vi "Load Hardware.vi"(8 "error in (no error)":errorcluster, 10 "Program only changes":bool=TRUE, 11 "Agilent ESG in":refnum<class "Agilent ESG.lvclass">) -> (0 "error out":errorcluster, 3 "Agilent ESG out":refnum<class "Agilent ESG.lvclass">)   [LabVIEW 2013, in "Agilent ESG.lvclass"]
uses:
  Agilent ESG.lvclass
  Agilent ESG.lvclass/Agilent ESG.ctl
panel:
  out "Hardware Image.Freq. [MHz]":dbl[](array[numeric])
  out "Last HWI Array":T1(array[cluster])
  out "Names encountered":string[](array[string])
  # "encapsulate HWI in cluser so each \"last encountered\"\ncan be a different length."
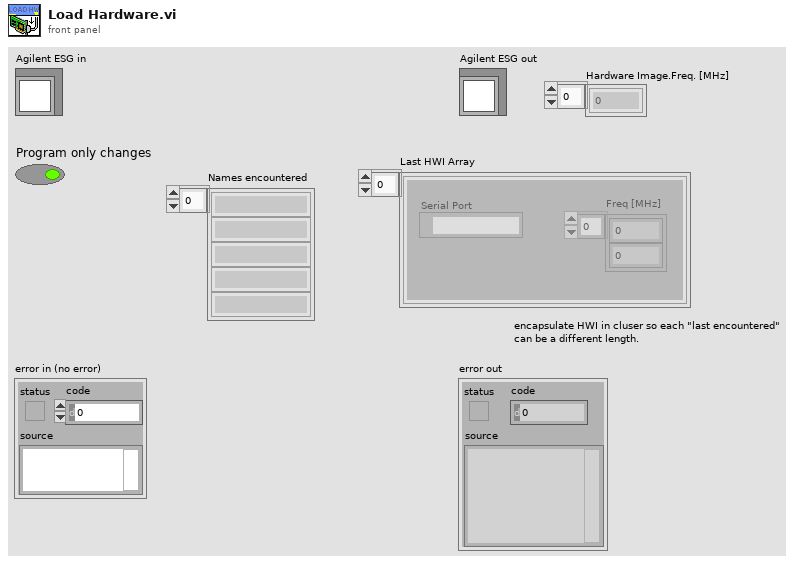
[diagram p1: front panel]
types:
  T1 = cluster{"Freq [MHz]":dbl[], "Serial Port":refnum<visa-resource-name>}[]
  T2 = enum16{"open", "replace", "create", "open or create", "replace or create", "replace or create with confirmation"}
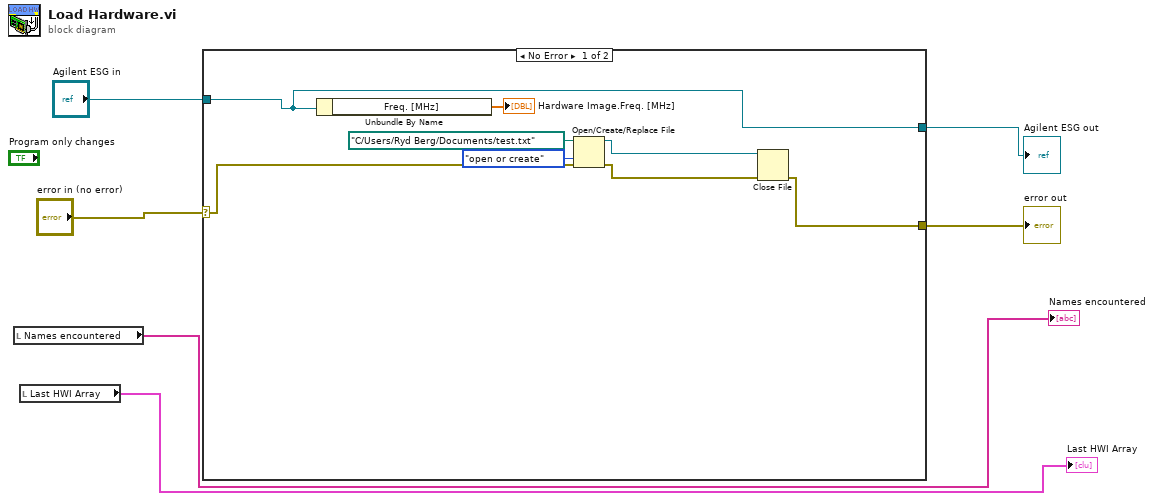
[diagram p0: block diagram]
diagram:
  n1 = local read "Names encountered"() -> (→"Names encountered":string[])
  n2 = local read "Last HWI Array"() -> (→"Last HWI Array":T1)
  n3 = case shown="No Error" "error in (no error)" {
    selector: "error in (no error)" -> [w13 w15]
    tunnel: "Agilent ESG in" -> [w11 w16]
    tunnel: [w12 w15] -> w2
    tunnel: [w11 w16] -> w1
    frame No Error {
      n4 = Unbundle By Name(w11) -> ("Freq. [MHz]"=→"Hardware Image.Freq. [MHz]":dbl[])
      n5 = Open/Create/Replace File(file path (use dialog)=path "C:/Users/Ryd Berg/Documents/test.txt", error in=w13, operation (0:open)=T2."open or create") -> (refnum out=w9:refnum<file>, error out=w8:errorcluster)  [unwired: 3 in, 1 out]
      n6 = Close File(refnum=w9, error in=w8) -> (error out=w12:errorcluster)  [unwired: 1 out]
    }
    frame Error {
    }
  }
  "error out" <- w2
  "Agilent ESG out" <- w1
